vi "3-FindMethods.vi"(3 "ProjectIndex":i32) -> ()   [LabVIEW 2016, in "TestVIs.lvlib"]
uses:
  TestVIs.lvlib
panel:
  out "Methods":cluster{"Class":string, "Array":string[]}[](array[cluster])
  out "Project-Name":string
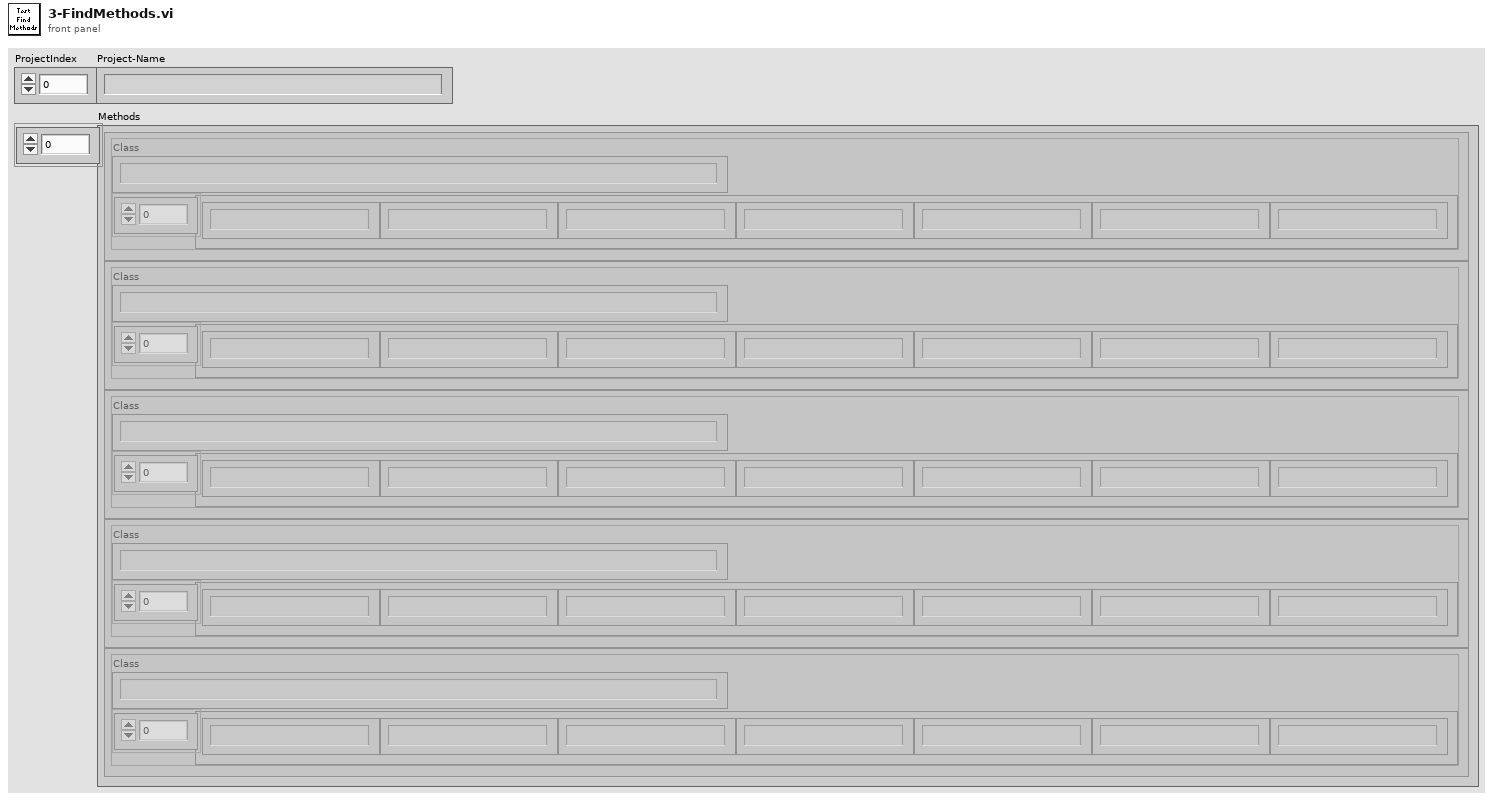
[diagram p1: front panel]
types:
  T1 = enum32{"invalid VI type", "Standard VI", "Control VI", "Global VI", "Polymorphic VI", "Configuration VI", "SubSystem", "Facade VI", "Method VI", "Statechart Diagram VI"}
  T2 = enum32{"invalid scope", "public", "private", "protected", "community"}
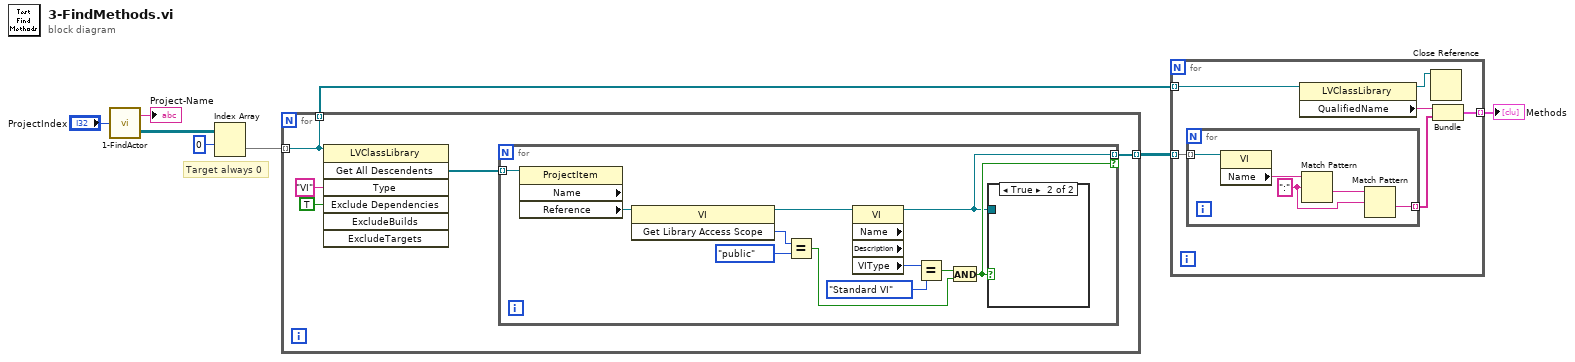
[diagram p0: block diagram]
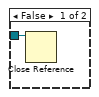
[diagram p2: hidden frame]
diagram:
  # "Target always 0"
  n1 = call "1-FindActor.vi"("ProjectIndex"="ProjectIndex") -> ("Actors"=w6:refnum<vi>[][], "Project-Name"=→"Project-Name":string)  [unwired: 2 in]
  n2 = Index Array(array=w6, index (row)=0) -> (element=w4:refnum<vi>[])  [unwired: 1 in]
  n3 = for {
    tunnel: w4 -> [w9] mode=indexing
    tunnel: [w10] -> w3 mode=indexing
    tunnel: [w9] -> w2 mode=indexing
    n4 = invoke class="LVClassLibrary" method="Get All Descendents"(reference=w9, "Type"="VI", "Exclude Dependencies"=TRUE ("ExcludeDependencies")) -> ("All Descendents"=w11:refnum<vi>[])  [unwired: 4 in, 6 out]
    n5 = for {
      tunnel: w11 -> [w23] mode=indexing
      tunnel: [w14] -> w10 mode=indexing if=w15
      n6 = property class="ProjectItem" props=["Name", "Reference"](reference=w23) -> ("Reference"=w24:refnum<vi>)  [unwired: 1 in, 3 out]
      n7 = invoke class="VI" method="Get Library Access Scope"(reference=w24) -> (reference out=w17:refnum<vi>, "Get Library Access Scope"=w21:T2)  [unwired: 2 in, 1 out]
      n8 = Equal?(x=w21, y=T2."public") -> (x = y?=w16:bool)
      n9 = property class="VI" props=["Name", "Description", "VIType"](reference=w17) -> (reference out=w14:refnum<vi>, "VIType"=w20:T1)  [unwired: 1 in, 3 out]
      n10 = Equal?(x=w20, y=T1."Standard VI") -> (x = y?=w19:bool)
      n11 = And(x=w19, y=w16) -> (x .and. y?=w15:bool)
      n12 = case shown="True" w15 {
        tunnel: w14 -> [w25 _]
        frame False {
          n13 = Close Reference(reference=w25) -> ()  [unwired: 1 in, 1 out]
        }
        frame True {
        }
      }
    }
  }
  n14 = for {
    tunnel: w3 -> [w31] mode=indexing
    tunnel: w2 -> [w30] mode=indexing
    tunnel: [w27] -> w1 mode=indexing
    n15 = for {
      tunnel: w31 -> [w36] mode=indexing
      tunnel: [w33] -> w28 mode=indexing
      w32 = ":" ("regular expression")
      n16 = property class="VI"(reference=w36) -> ("Name"=w35:string)  [unwired: 1 in, 2 out]
      n17 = Match Pattern(string=w35, regular expression=w32) -> (after substring=w34:string)  [unwired: 1 in, 3 out]
      n18 = Match Pattern(string=w34, regular expression=w32) -> (after substring=w33:string)  [unwired: 1 in, 3 out]
    }
    n19 = property class="LVClassLibrary"(reference=w30) -> (reference out=w26:refnum<vi>, "QualifiedName"=w29:string)  [unwired: 1 in, 1 out]
    n20 = Close Reference(reference=w26) -> ()  [unwired: 1 in, 1 out]
    n21 = Bundle("QualifiedName"=w29, w28) -> (w27:cluster{"QualifiedName":string, string[]})  [unwired: 1 in]
  }
  "Methods" <- w1
